vi "niRFUtil WFM Replace Pt by Pt (complex array).vi"(0 "Complex Array In":T1 format="%.2f", 1 "Replace Index":i32, 2 "Replace With":T1 format="%.2f", 3 "Default Value (0)":sgl=-inf min=0 max=127 format="%.2f") -> (5 "Complex Array Out":T1 format="%.2f")   [LabVIEW 2015, in "niRFUtil.lvlib"]
uses:
  niRFUtil.lvlib
  Includes/niRFUtil INC Complex Array.ctl
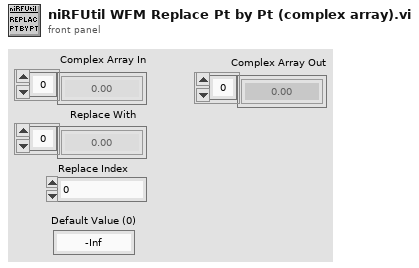
[diagram p1: front panel]
types:
  T1 = typedef "niRFUtil.lvlib/niRFUtil INC Complex Array.ctl" = csg[]
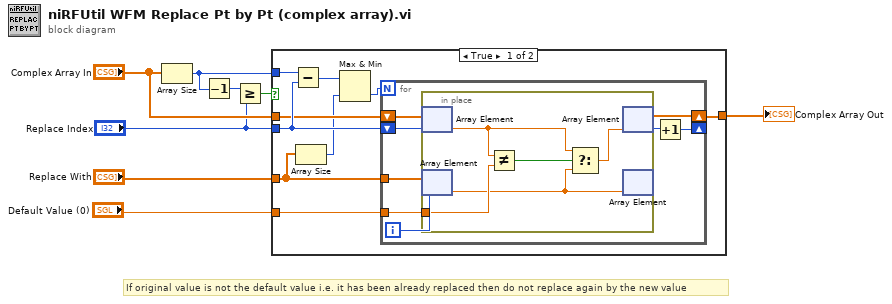
[diagram p0: block diagram]
diagram:
  # "If original value is not the default value i.e. it has been already replaced then do not replace again by the new value"
  n1 = Array Size(array="Complex Array In") -> (size(s)=w8:i32)
  n2 = Decrement(x=w8) -> (x-1=w7:i32)
  n3 = Greater Or Equal?(x=w7, y="Replace Index") -> (x >= y?=w6:bool)
  n4 = case shown="True" w6 {
    tunnel: "Complex Array In" -> [w16 w31]
    tunnel: [w10 w31] -> w2
    tunnel: "Replace With" -> [w14 _]
    tunnel: "Replace Index" -> [w17 _]
    tunnel: w8 -> [w15 _]
    tunnel: "Default Value (0)" -> [w9 _]
    frame True {
      n5 = Subtract(x=w15, y=w17) -> (x-y=w13:i32)
      n6 = Array Size(array=w14) -> (size(s)=w12:i32)
      n7 = Max & Min(x=w13, y=w12) -> (min(x,y)=w11:i32)  [unwired: 1 out]
      n8 = for {
        N: w11 -> [_]
        shift-right: [w19] -> _
        shift-left: w17 -> [w24]
        shift-right: [w20] -> w10
        shift-left: w16 -> [w25]
        tunnel: w14 -> [w23]
        tunnel: w9 -> [w18]
        i -> [w22]
        n9 = in-place {
          in-place-border: w18 -> [w29]
          n10 = in-place-array #1(w25, w24) -> (w28:csg)
          n11 = in-place-array #2(w23, w22) -> (w26:csg)
          n12 = Not Equal?(x=w28, y=w29) -> (x != y?=w27:bool)
          n13 = Select(t=w28, s=w27, f=w26) -> (s? t:f=w30:csg)
          n14 = in-place-array #1(w30) -> (w20:T1, w21:i32)
          n15 = in-place-array #2(w26) -> ()  [unwired: 2 out]
        }
        n16 = Increment(x=w21) -> (x+1=w19:i32)
      }
    }
    frame False {
    }
  }
  "Complex Array Out" <- w2
